vi "Ultrasonic Monitor.vi"   [LabVIEW 2014]
uses:
  Ultrasonic Data.vi
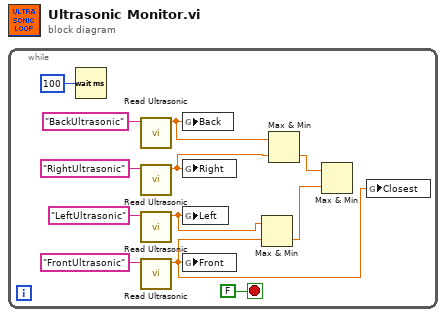
[diagram p0: block diagram]
diagram:
  n1 = while {
    stop <- FALSE stop-if-true
    n2 = Wait (ms)(milliseconds to wait=u32 100) -> ()  [unwired: 1 out]
    n3 = call "Read Ultrasonic.vi"("ultrasonic name"="BackUltrasonic") -> ("Range"=w6:dbl)  [unwired: 10 in]
    n4 = call "Read Ultrasonic.vi"("ultrasonic name"="RightUltrasonic") -> ("Range"=w5:dbl)  [unwired: 10 in]
    n5 = call "Read Ultrasonic.vi"("ultrasonic name"="LeftUltrasonic") -> ("Range"=w4:dbl)  [unwired: 10 in]
    n6 = call "Read Ultrasonic.vi"("ultrasonic name"="FrontUltrasonic") -> ("Range"=w1:dbl)  [unwired: 10 in]
    n7 = global write "Ultrasonic Data.vi" "Back"(w6) -> ()
    n8 = global write "Ultrasonic Data.vi" "Right"(w5) -> ()
    n9 = global write "Ultrasonic Data.vi" "Left"(w4) -> ()
    n10 = global write "Ultrasonic Data.vi" "Front"(w1) -> ()
    n11 = Max & Min(x=w4, y=w1) -> (min(x,y)=w2:dbl)  [unwired: 1 out]
    n12 = Max & Min(x=w6, y=w5) -> (min(x,y)=w3:dbl)  [unwired: 1 out]
    n13 = Max & Min(x=w3, y=w2) -> ()  [unwired: 2 out]
    n14 = global write "Ultrasonic Data.vi" "Closest"(w1) -> ()
  }
